vi "Partial Cluster With Array Of Analog Waveform.vi"(8 "LV Control Name Paths":string[](array[string]), 9 "TS Variable Name Paths":string[](array[string]), 10 "Sequence Context":refnum<k7>, 11 "Cluster":cluster{"Numeric":dbl, "Array":waveform(dbl)[]}={"Numeric"=0.0, "Array"=[{"t0"=timestamp(0 s since 1904-01-01), "dt"=0.0, "Y"=[]}]}) -> (0 "error out":errorcluster, 1 "Report Text":string, 2 "PASS/FAIL Flag":bool, 3 "Cluster 2":cluster{"Numeric":dbl, "Array":waveform(dbl)[]})   [LabVIEW 2011]
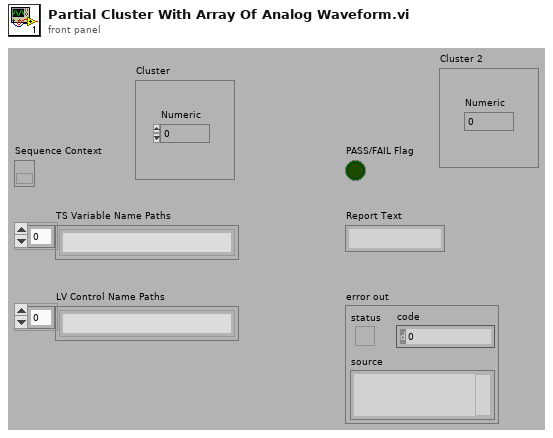
[diagram p1: front panel]
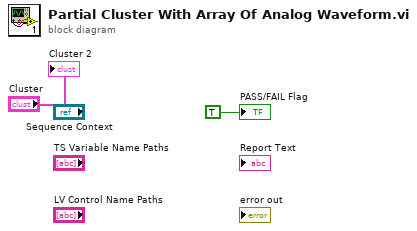
[diagram p0: block diagram]
diagram:
  "PASS/FAIL Flag" <- TRUE ("PASS/FAIL Flag")
  "Cluster 2" <- "Cluster"
